vi "Hardware-ExpansionRIO.vi"(11 "DSI Reference":refnum<class "DCM-DSI.lvclass">) -> ()   [LabVIEW 2016, in "DSI-RT.lvlib"]
uses:
  DSI-RT.lvlib
  Classes/DCM-DSI/DCM-DSI.lvclass
  Shared/Typedefs/System-ExpansionRIO-State.ctl
  <vilib>/Powertrain Controls/Device Drivers/DCM/Rev0/RT/DCM - RT.lvclass/DCM - RT.ctl
  <vilib>/Powertrain Controls/Device Drivers/DCM/Rev0/RT/Read Stop Target.vi
  Classes/DCM-DSI/Read DCM Ref.vi
  Classes/DCM-DSI/Write ExpansionRIO.vi
  Classes/DCM-DSI/Read ExpansionRIO.vi
  <vilib>/FPGAPlugInAG/Dynamic/niLvFpga_Close_Dynamic.vi
  <vilib>/Powertrain Controls/Device Drivers/DCM/Rev0/RT/DCM - RT.lvclass
  <vilib>/addons/Software Calibration Management/xSCM/CalPoint.xnode
  <vilib>/rvi/interface/nirviCloseFPGA/nirviCloseFPGA.xnode
  <vilib>/addons/Software Calibration Management/xSCM/ni_scm.dll
  Shared/DSI-Shared.lvlib
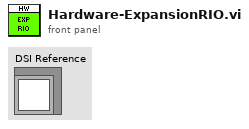
[diagram p1: front panel]
types:
  T1 = typedef "DSI-Shared.lvlib/System-ExpansionRIO-State.ctl" = cluster{"Error":bool, "Description":string}
  T2 = cluster{"Enable Expansion RIO":bool, "Bitfile":enum16{"Standard (NI 9149)", "Custom"}, "IP Address":string, "Custom Bitfile Path":string}
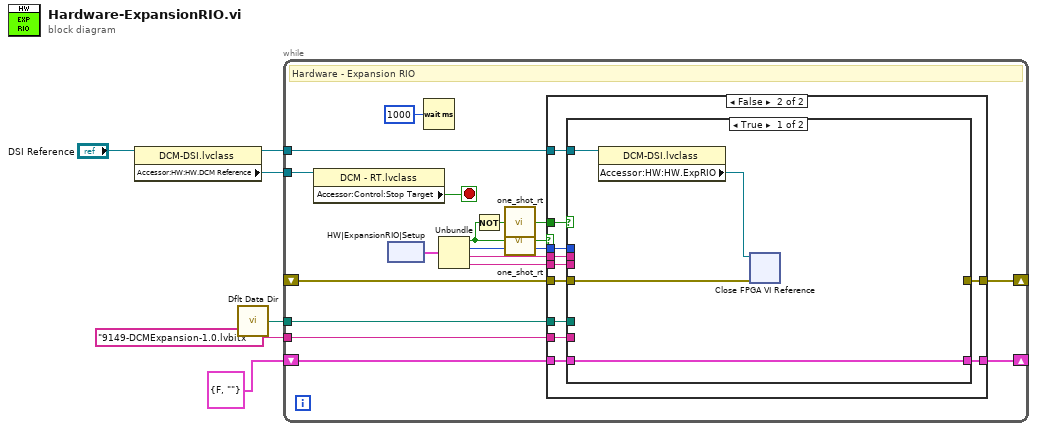
[diagram p0: block diagram]
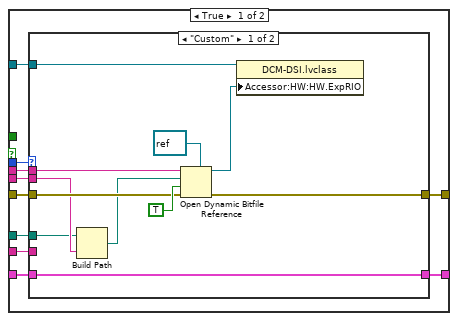
[diagram p2: hidden frame]
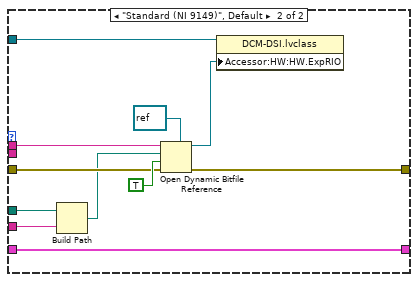
[diagram p3: hidden frame]
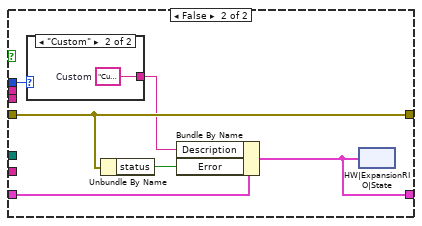
[diagram p4: hidden frame]
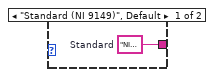
[diagram p5: hidden frame]
diagram:
  n1 = property class="DCM-DSI.lvclass"(reference="DSI Reference") -> (reference out=w4:refnum<class "DCM-DSI.lvclass">, "Accessor:HW:HW.DCM Reference"=w5:refnum<class "DCM - RT.lvclass">)  [unwired: 1 in, 1 out]
  n2 = call <vilib>:"Dflt Data Dir.vi"() -> ("App:Default Data Directory"=w3:path)
  n3 = while {
    tunnel: w5 -> [w24]
    tunnel: w4 -> [w12]
    shift-right: [w18] -> _
    shift-left: _ -> [w17]
    tunnel: w3 -> [w16]
    tunnel: "9149-DCMExpansion-1.0.lvbitx" ("name or relative path") -> [w15]
    shift-right: [w9] -> _
    shift-left: T1 {"Error"=FALSE, "Description"=""} ("ExpansionRIOStatus") -> [w10]
    stop <- w23 stop-if-true
    # "Hardware - Expansion RIO"
    n4 = property class="DCM - RT.lvclass"(reference=w24) -> ("Accessor:Control:Stop Target"=w23:bool)  [unwired: 1 in, 2 out]
    n5 = xnode "HW|ExpansionRIO|Setup"() -> ("Value"=w22:T2)
    n6 = Wait (ms)(milliseconds to wait=u32 1000) -> ()  [unwired: 1 out]
    n7 = Unbundle(w22) -> ("Enable Expansion RIO"=w14:bool, "Bitfile"=w21:enum16{"Standard (NI 9149)", "Custom"}, "IP Address"=w20:string, "Custom Bitfile Path"=w19:string)
    n8 = Not(x=w14) -> (.not. x?=w13:bool)
    n9 = call <vilib>:"one_shot_rt.vi"("I"=w13) -> ("O"=w11:bool)
    n10 = call <vilib>:"one_shot_rt.vi"("I"=w14) -> ("O"=w8:bool)
    n11 = case shown="False" w8 {
      tunnel: w21 -> [w34 w57]
      tunnel: w20 -> [w33 w67]
      tunnel: w19 -> [w32 w66]
      tunnel: [w31 w65] -> w18
      tunnel: w16 -> [w30 w64]
      tunnel: w17 -> [w29 w63]
      tunnel: w15 -> [w28 w62]
      tunnel: w12 -> [w27 w61]
      tunnel: w11 -> [_ w60]
      tunnel: w10 -> [w26 w59]
      tunnel: [w25 w58] -> w9
      frame True {
        n12 = case shown="\"Custom\"" w34 {
          tunnel: w33 -> [w45 w56]
          tunnel: w32 -> [w41 _]
          tunnel: [w36 w47] -> w31
          tunnel: w30 -> [w39 w51]
          tunnel: w29 -> [w42 w53]
          tunnel: w28 -> [_ w50]
          tunnel: w27 -> [w38 w49]
          tunnel: [w35 w46] -> w25
          tunnel: w26 -> [w35 w46]
          frame "Custom" {
            n13 = Build Path(base path=w39, name or relative path=w41) -> (appended path=w40:path)
            n14 = Open Dynamic Bitfile Reference(0:w45, 1:w40, 2:TRUE ("Run When Loaded"), 3:w42, 4:refnum<k20> refnum ("Type")) -> (5:w37:refnum<k20>, 8:w36:errorcluster)
            n15 = property class="DCM-DSI.lvclass"(reference=w38, "Accessor:HW:HW.ExpRIO"=w37) -> ()  [unwired: 1 in, 2 out]
          }
          frame "Standard (NI 9149)", Default {
            n16 = Build Path(base path=w51, name or relative path=w50) -> (appended path=w52:path)
            n17 = Open Dynamic Bitfile Reference(0:w56, 1:w52, 2:TRUE ("Run When Loaded"), 3:w53, 4:refnum<k20> refnum ("Type")) -> (5:w48:refnum<k20>, 8:w47:errorcluster)
            n18 = property class="DCM-DSI.lvclass"(reference=w49, "Accessor:HW:HW.ExpRIO"=w48) -> ()  [unwired: 1 in, 2 out]
          }
        }
      }
      frame False {
        n19 = case shown="True" w60 {
          tunnel: w67 -> [_ _]
          tunnel: w66 -> [_ _]
          tunnel: [_ w76] -> w65
          tunnel: w64 -> [_ _]
          tunnel: w63 -> [w70 w76]
          tunnel: w62 -> [_ _]
          tunnel: w61 -> [w71 _]
          tunnel: w59 -> [w68 w75]
          tunnel: [w68 w72] -> w58
          tunnel: w57 -> [_ w74]
          frame True {
            n20 = property class="DCM-DSI.lvclass"(reference=w71) -> ("Accessor:HW:HW.ExpRIO"=w69:refnum<k20>)  [unwired: 1 in, 2 out]
            n21 = xnode ("Close FPGA VI Reference")("FPGA VI Reference In"=w69, "error in"=w70) -> ()  [unwired: 1 out]
          }
          frame False {
            n22 = case shown="\"Custom\"" w74 {
              tunnel: [w83 w84] -> w73
              frame "Standard (NI 9149)", Default {
                w83 = "NI 9419 EthernetRIO, 6x VR/Hall channels, 2x wide-band O2 sensors,  and 16x ESTTL channels.  For more information about extending DCM DSI I/O capabilities, consult the DCM DSI User's Manual."  # Standard
              }
              frame "Custom" {
                w84 = "Custom bitfile.  For more information about extending DCM DSI I/O capabilities, consult the DCM DSI User's Manual."  # Custom
              }
            }
            n23 = Unbundle By Name(w76) -> ("status"=w77:bool)
            n24 = Bundle By Name(cluster=w75, "Description"=w73, "Error"=w77) -> (w72:T1)
            n25 = xnode "HW|ExpansionRIO|State"("Value"=w72) -> ()
          }
        }
      }
    }
  }
